vi "2 mission_interpreter.vi"(8 "error in (no error)":errorcluster) -> (0 "error out":errorcluster)   [LabVIEW 2011]
doc: "Handles mission status. If the previous mission is complete or nonexistent, we log that info, and Start the next mission from the Mission Queue. If the mission is not complete, we call the Update Waypoints method on that mission to check the needs of the individual mission."
uses:
  2 Classes/Missions/GenericMission/GenericMission.lvclass
  2 Globals/2 Global.vi
  2 Globals/2 Message Logger.vi
  2 Classes/MissionQueue/MissionQueue.lvclass
  2 Classes/Logger/Logger.lvclass
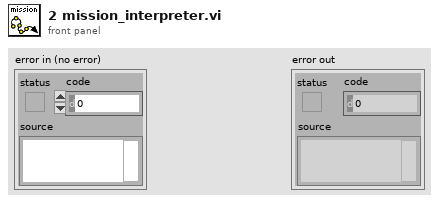
[diagram p1: front panel]
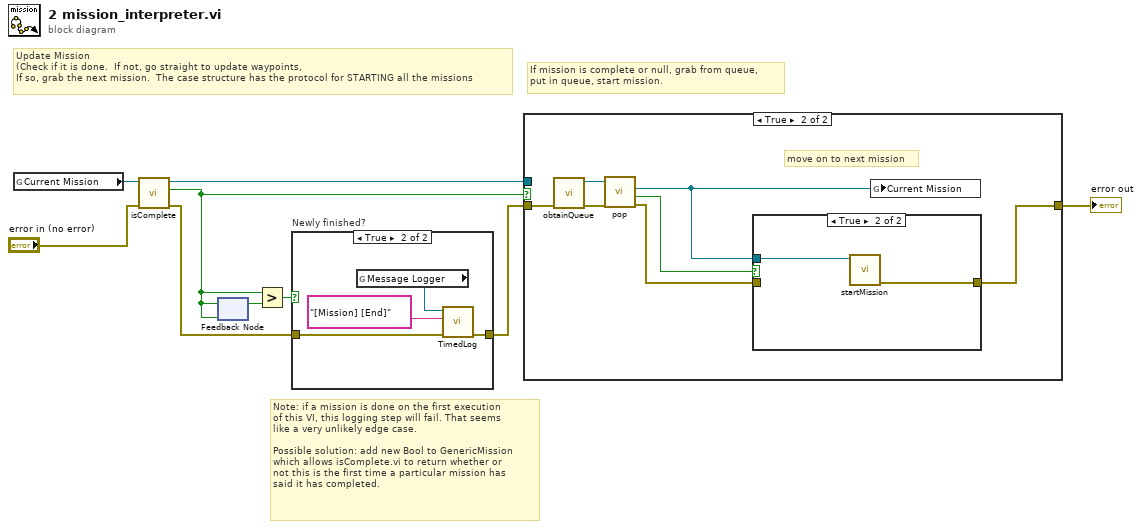
[diagram p0: block diagram]
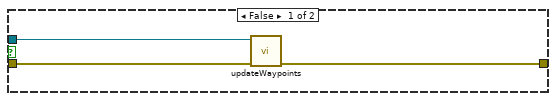
[diagram p3: hidden frame]
diagram:
  # "Note: if a mission is done on the first execution\nof this VI, this logging step will fail. That seems\nlike a very unlikely edge case.\n\nPossible solution: add new Bool to GenericMission\nwhich allows isComplete.vi to return whether or\nnot this is the first time a particular mission has\nsaid it has completed."
  # "Update Mission\n(Check if it is done.  If not, go straight to update waypoints,\nIf so, grab the next mission.  The case structure has the protocol for STARTING all the missions"
  # "If mission is complete or null, grab from queue, \nput in queue, start mission."
  n1 = global read "2 Global.vi" "Current Mission"() -> (w9:refnum<class "GenericMission.lvclass">)
  n2 = call-dynamic "isComplete.vi"("error in (no error)"="error in (no error)", "Mission in"=w9) -> ("error out"=w2:errorcluster, "Mission Complete?"=w5:bool, "Mission out"=w8:refnum<class "GenericMission.lvclass">)  [unwired: 7 in]
  n3 = feedback-in #1(w5) -> ()
  n4 = feedback #1(w5) -> (w4:bool)
  n5 = Greater?(x=w5, y=w4) -> (0:w3:bool)
  n6 = case "Newly finished?" shown="True" w3 {
    tunnel: w2 -> [w10 w12]
    tunnel: [w10 w11] -> w1
    frame False {
    }
    frame True {
      n7 = global read "2 Message Logger.vi" "Message Logger"() -> (w13:refnum<class "Logger.lvclass">)
      n8 = call "TimedLog.vi"("error in (no error)"=w12, "Message"="[Mission] [End]", "Logger in"=w13) -> ("error out"=w11:errorcluster)  [unwired: 6 in, 2 out]
    }
  }
  n9 = case shown="True" w5 {
    tunnel: w8 -> [w17 _]
    tunnel: w1 -> [w16 w19]
    tunnel: [w15 w20] -> w6
    frame False {
      n10 = call-dynamic "updateWaypoints.vi"("error in (no error)"=w16, "GenericMission in"=w17) -> ("error out"=w15:errorcluster)  [unwired: 8 in, 1 out]
    }
    frame True {
      # "move on to next mission"
      n11 = call "obtainQueue.vi"("Error In"=w19) -> ("Error Out"=w21:errorcluster, "MissionQueue.lvclass"=w23:refnum<class "MissionQueue.lvclass">)  [unwired: 9 in]
      n12 = call "pop.vi"("error in (no error)"=w21, "MissionQueue in"=w23) -> ("error out"=w18:errorcluster, "Valid?"=w24:bool, "GenericMission.lvclass"=w22:refnum<class "GenericMission.lvclass">)  [unwired: 6 in, 1 out]
      n13 = case shown="True" w24 {
        tunnel: w22 -> [_ w26]
        tunnel: w18 -> [w25 _]
        tunnel: [w25 w27] -> w20
        frame False {
          # "no more valid missions."
        }
        frame True {
          n14 = call-dynamic "startMission.vi"("GenericMission in"=w26) -> ("error out"=w27:errorcluster)  [unwired: 9 in, 1 out]
        }
      }
      n15 = global write "2 Global.vi" "Current Mission"(w22) -> ()
    }
  }
  "error out" <- w6
